vi "MicroStruct-XY-abs.vi"() -> ()   [LabVIEW 2014]
doc: "Newport Motion Controler\nThis program make lines structure\n\nAndré Romero - 2020\nandretec@ifsc.usp.br"
uses:
  <vilib>/Platform/TimedLoop/XDataNode/timing_clust.ctl
  <vilib>/Platform/TimedLoop/XDataNode/nitl_modes.ctl
  <vilib>/Platform/TimedLoop/XDataNode/wakeup.ctl
  Basic-VIs/Global Motor Axis.vi
  <vilib>/Platform/TimedLoop/XDataNode/XDataNode.xnode
  <userlib>/Newport ESP301/Newport ESP301.lvlib
  <vilib>/Platform/TimedLoop/XDataNode/XDNodeRunTimeDep.lvlib
panel:
  in  "Swap motor":bool
  out "XY Graph":cluster{dbl[], dbl[]}(graph)={[0.0, 0.0, 0.0345, 0.108, 0.2205, 0.3735, 0.564, 0.7665, 0.964, 1.0005, 1.0, 0.9995, 0.9995, 0.9815, 0.9225, 0.8235, 0.686, 0.505, 0.308, 0.108, -0.002, 0.0, 0.0005, 0.0, 0.012, 0.066, 0.1575, 0.2915, 0.465, 0.6645, 0.866, 1.0025, 1.0, 1.0, 0.9995, 0.9965, 0.9565, 0.8775, 0.7585, 0.6, 0.4055, 0.204, 0.006, -0.0005, 0.0005, 0.0, 0.0005, 0.0345, 0.108, 0.2215, 0.375, 0.566, 0.7675, 0.9685, 1.001, 1.0, 1.0, 0.9995, 0.9855, 0.9315, 0.8375, 0.7035, 0.5295, 0.331, 0.1305, -0.0025, 0.0, 0.0005, 0.0, 0.009, 0.0585, 0.148, 0.2765, 0.4475, 0.645, 0.8435, 1.003, 1.0005, 1.0, 0.9995, 0.999, 0.9625, 0.887, 0.773, 0.6175, 0.4265, 0.225, 0.028, -0.0005, 0.0005, 0.0, 0.0005, 0.031, 0.1025, 0.2125, 0.364, 0.55, 0.751, 0.9525, 1.001, 1.0, 1.0, 0.9995, 0.986, 0.9315, 0.8385, 0.705, 0.531, 0.3315, 0.1305, -0.002, 0.0, 0.0005, 0.0, 0.0085, 0.057, 0.146, 0.2735, 0.44, 0.6395, 0.8415, 1.003, 1.0, 1.0, 1.0, 0.9995, 0.9645, 0.891, 0.7775, 0.6255, 0.4355, 0.2345, 0.033, -0.0005, 0.0005, 0.0, 0.0, 0.0185, 0.0775, 0.1765, 0.3145, 0.4925, 0.6925, 0.895, 1.002, 1.0, 1.0, 0.9995, 0.9865, 0.933, 0.839, 0.7055, 0.535, 0.333, 0.1325, -0.0025, 0.0, 0.0005, 0.0, 0.0025, 0.043, 0.1225, 0.2425, 0.4015, 0.5945, 0.795, 0.9955, 1.0005, 1.0, 1.0, 0.9995, 0.965, 0.8915, 0.7775, 0.625, 0.4335, 0.235, 0.035, -0.0005, 0.0005, 0.0, 0.0, 0.0185, 0.078, 0.176, 0.3155, 0.4925, 0.693, 0.892, 1.002, 1.0, 1.0, 0.9995, 0.9865, 0.933, 0.8405, 0.706, 0.5345, 0.3325, 0.1335, -0.0025, 0.0, 0.0005, 0.0, 0.002, 0.043, 0.1225, 0.2415, 0.401, 0.594, 0.7955, 0.9945, 1.0005, 1.0, 0.9995, 0.9995, 0.9655, 0.891, 0.7775, 0.623, 0.431, 0.233, 0.032, 0.0, 0.0005, 0.0, 0.0], [0.0, 0.0, 0.0, 0.0, 0.0, 0.0, 0.0, 0.0, 0.0, 0.0, 0.021, 0.0825, 0.1015, 0.101, 0.1005, 0.1, 0.1, 0.1, 0.1, 0.1, 0.1, 0.104, 0.158, 0.2015, 0.2015, 0.2005, 0.2, 0.2, 0.2, 0.2, 0.2, 0.2, 0.2, 0.2425, 0.3015, 0.3015, 0.301, 0.3005, 0.3, 0.3, 0.3, 0.3, 0.3, 0.3, 0.328, 0.3975, 0.4015, 0.401, 0.4005, 0.4, 0.4, 0.4, 0.4, 0.4, 0.4, 0.411, 0.468, 0.5015, 0.501, 0.5005, 0.5, 0.5, 0.5, 0.5, 0.5, 0.5, 0.504, 0.557, 0.6015, 0.601, 0.6005, 0.6, 0.6, 0.6, 0.6, 0.6, 0.6, 0.6, 0.6365, 0.7015, 0.7015, 0.701, 0.7, 0.7, 0.7, 0.7, 0.7, 0.7, 0.7, 0.7275, 0.7955, 0.8015, 0.801, 0.8005, 0.8, 0.8, 0.8, 0.8, 0.8, 0.8, 0.8105, 0.868, 0.902, 0.9015, 0.9, 0.9, 0.9, 0.9, 0.9, 0.9, 0.9, 0.9005, 0.9485, 1.0015, 1.0015, 1.0005, 1.0, 1.0, 1.0, 0.9995, 0.9995, 1.0, 1.0, 1.0345, 1.1015, 1.1015, 1.101, 1.1, 1.1, 1.1, 1.1, 1.1, 1.1, 1.1, 1.128, 1.1865, 1.2015, 1.201, 1.2, 1.2, 1.2, 1.1995, 1.2, 1.2, 1.2, 1.207, 1.259, 1.3015, 1.3015, 1.3005, 1.3, 1.3, 1.3, 1.3, 1.3, 1.3, 1.3, 1.343, 1.4015, 1.4015, 1.4005, 1.4, 1.4, 1.4, 1.4, 1.3995, 1.3995, 1.4, 1.429, 1.4985, 1.5015, 1.5005, 1.5, 1.5, 1.5, 1.5, 1.5, 1.5, 1.5, 1.5175, 1.578, 1.6015, 1.601, 1.6005, 1.6, 1.6, 1.6, 1.6, 1.6, 1.6, 1.605, 1.659, 1.7015, 1.701, 1.7005, 1.7, 1.7, 1.7, 1.7, 1.7, 1.7, 1.7, 1.7425, 1.802, 1.8015, 1.8005, 1.8, 1.8, 1.8, 1.8, 1.8, 1.8, 1.8, 1.8295, 1.8995, 1.9015, 1.9005, 1.9, 1.9, 1.9, 1.9, 1.9, 1.8995, 1.8995, 1.918, 1.979, 2.002]}
  in  "N Cycles":i32=10 min=1
  in  "Acceleration (0 units/s²)":dbl=1.0 min=0.0 format="%#.4g"
  in  "Velocity (units/s)":dbl=1.0 min=0.0 format="%#.4g"
  in  "d (mm)":dbl=0.1
  in  "L (mm)":dbl=1.0
  out "X Position (mm)":dbl format="%.6g"
  out "Y Position (mm)":dbl=2.002 format="%.6g"
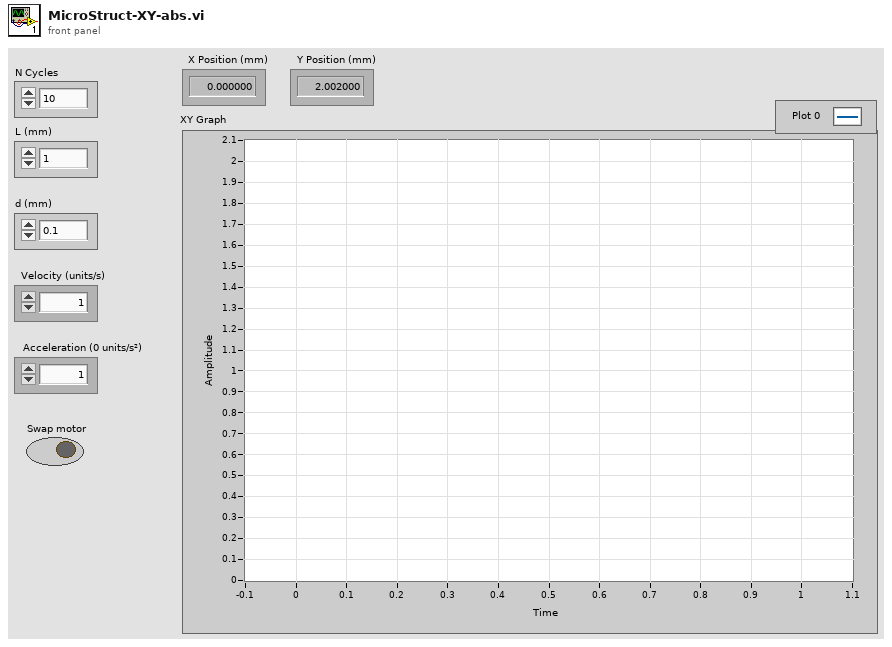
[diagram p1: front panel]
types:
  T1 = typedef "XDNodeRunTimeDep.lvlib/timing_clust.ctl" = cluster{"Expected End [f-1]":u64, "Actual End [f-1]":u64, "Finished Late? [f-1]":bool, "Expected End [i-1]":u64, "Actual End [i-1]":u64, "Finished Late? [i-1]":bool, "Expected Start [i]":u64, "Actual Start [i]":u64, "Expected Start [f]":u64, "Actual Start [f]":u64, "Source Name":string, "Structure Name":string, "Period":i64, "Deadline":i64, "Offset":i64, "Start":i64, "Priority":i32, "Timeout":i32, "Mode":T2, "Wakeup Reason":T3, "Error":errorcluster, "Source Type":string, "Secondary Source Type":string, "Global End Time":u64, "Global Start Time":u64, "Frame Duration":u64, "Iteration Duration":u64, "Assigned CPU":i32, "I/O Scan Engine Mode":u32}
  T2 = typedef "XDNodeRunTimeDep.lvlib/nitl_modes.ctl" = enum32{"No Change", "Process missed periods, maintain original phase", "Discard missed periods, maintain original phase", "Process missed periods, ignore original phase", "Discard missed periods, ignore original phase"}
  T3 = typedef "XDNodeRunTimeDep.lvlib/wakeup.ctl" = enum32{"Normal", "Aborted", "Asynchronous wakeup", "Timing source error", "Timed loop error", "Timeout"}
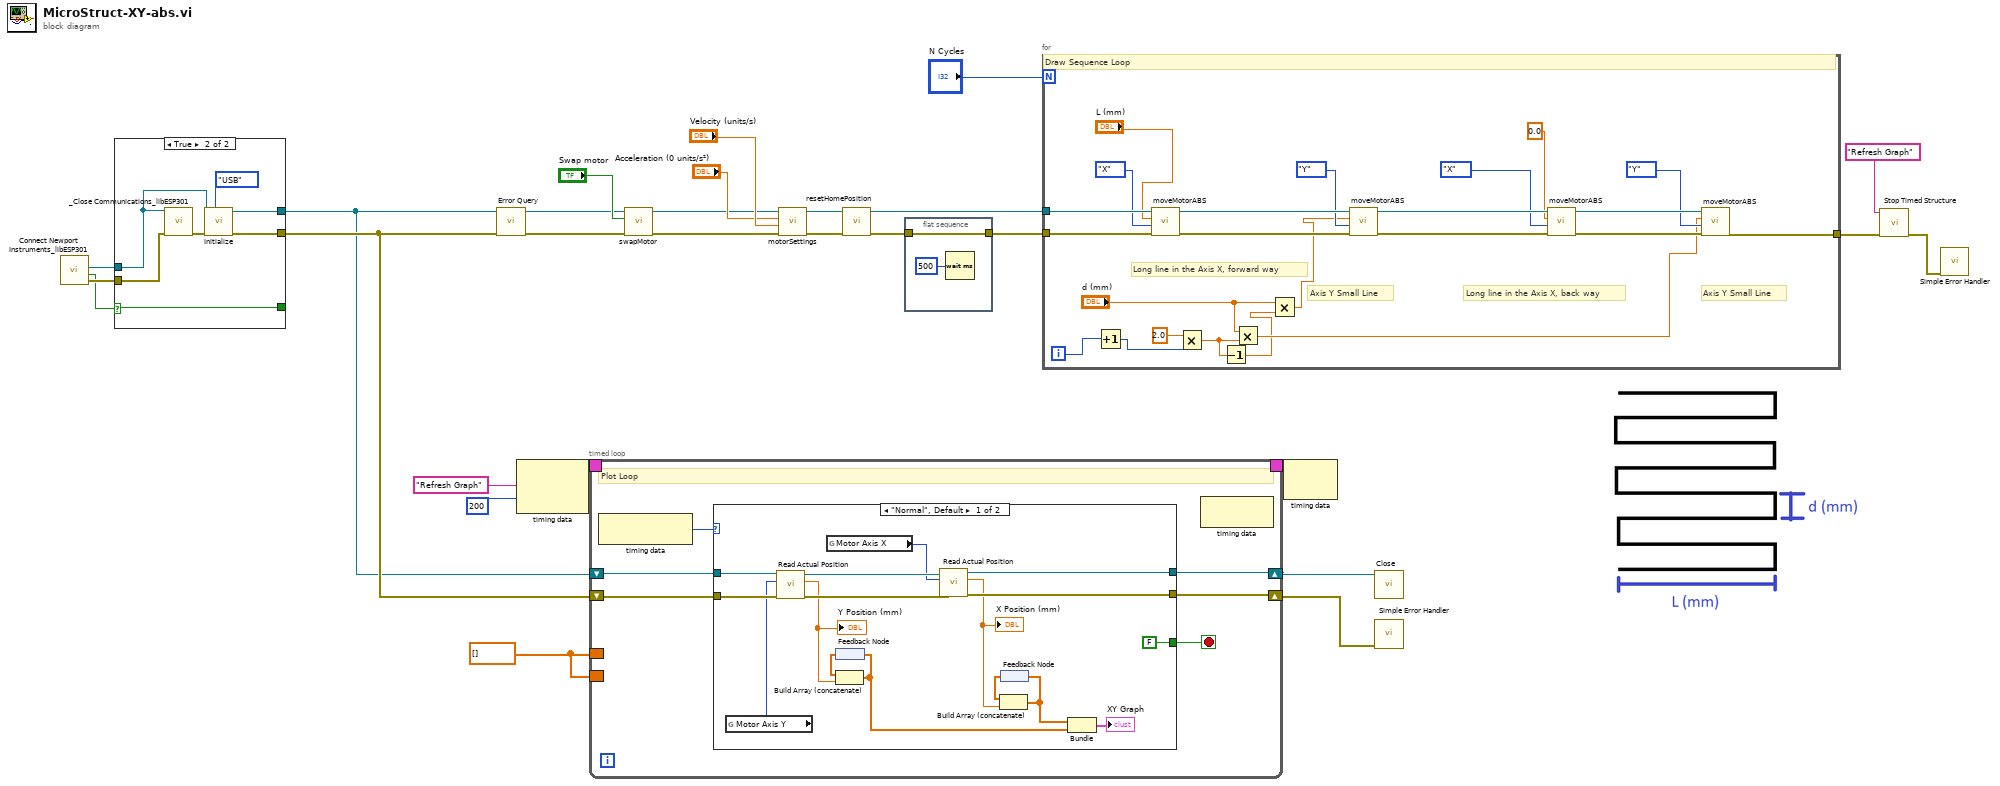
[diagram p0: block diagram]
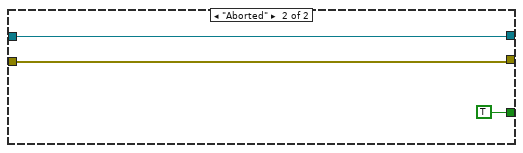
[diagram p2: hidden frame]
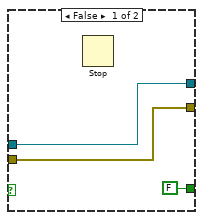
[diagram p3: hidden frame]
diagram:
  w13 = dbl[] []
  n1 = call <userlib>:"Connect Newport Instruments_libESP301.vi"() -> ("error (duplicate)"=w28:errorcluster, "Connected"=w22:bool, "VISA resource name (duplicate)"=w27:refnum<visa-resource-name>)  [unwired: 7 in, 2 out]
  n2 = case shown="True" w22 {
    selector: w22 -> [_ w32]
    tunnel: w28 -> [w29 w36]
    tunnel: w27 -> [w30 w35]
    tunnel: [w29 w34] -> w26
    tunnel: [w30 w33] -> w25
    tunnel: [FALSE w32] -> _
    frame False {
      n3 = Stop() -> ()  [unwired: 1 in]
    }
    frame True {
      n4 = call <userlib>:"_Close Communications_libESP301.vi"("Instrument Channel"=w35, "error in (no error)"=w36) -> ("error out"=w38:errorcluster)  [unwired: 13 in]
      n5 = call <userlib>:"Initialize.vi"("VISA resource name"=w35, "error in (no error)"=w38, "Serial Link (RS232)"=enum16{"RS232", "USB"}."USB") -> ("VISA resource name out"=w33:refnum<visa-resource-name>, "error out"=w34:errorcluster)  [unwired: 6 in]
    }
  }
  n6 = call <userlib>:"Error Query.vi"("error in (no error)"=w26, "VISA resource name"=w25) -> ("error out"=w8:errorcluster, "VISA resource name out"=w9:refnum<visa-resource-name>)  [unwired: 2 in, 2 out]
  n7 = node-c288("Refresh Graph" ("Structure Name"), i64 200 ("Period")) -> (w21:T1)
  n8 = timed-loop {
    timing: w21 -> [_]
    timing-out: [_] -> w20
    shift-right: [w42] -> w24
    shift-left: w25 -> [w44]
    shift-right: [w41] -> w23
    shift-left: w26 -> [w43]
    border: w13 -> [_]
    border: w13 -> [_]
    stop <- w39 stop-if-true
    # "Plot Loop"
    n9 = node-c288() -> (w40:T3)  [unwired: 1 in]
    n10 = case shown="\"Normal\", Default" w40 {
      tunnel: w44 -> [w60 w62]
      tunnel: w43 -> [w59 w61]
      tunnel: [w56 w62] -> w42
      tunnel: [w55 w61] -> w41
      tunnel: [FALSE TRUE] -> w39
      frame "Normal", Default {
        n11 = global read "Global Motor Axis.vi" "Motor Axis Y"() -> (w45:i32)
        n12 = call <userlib>:"Read Actual Position.vi"("error in (no error)"=w59, "Axis (1)"=w45, "VISA resource name"=w60) -> ("error out"=w57:errorcluster, "Position (units)"=w50:dbl, "VISA resource name out"=w58:refnum<visa-resource-name>)  [unwired: 2 in]
        "Y Position (mm)" <- w50
        n13 = global read "Global Motor Axis.vi" "Motor Axis X"() -> (w46:i32)
        n14 = feedback #1() -> (w53:dbl[])
        n15 = Build Array (concatenate)(w53, w50) -> (w48:dbl[])
        n16 = feedback-in #1(w48) -> ()
        n17 = call <userlib>:"Read Actual Position.vi"("error in (no error)"=w57, "Axis (1)"=w46, "VISA resource name"=w58) -> ("error out"=w55:errorcluster, "Position (units)"=w51:dbl, "VISA resource name out"=w56:refnum<visa-resource-name>)  [unwired: 2 in]
        "X Position (mm)" <- w51
        n18 = feedback #2() -> (w52:dbl[])
        n19 = Build Array (concatenate)(w52, w51) -> (w49:dbl[])
        n20 = feedback-in #2(w49) -> ()
        n21 = Bundle(w49, w48) -> (→"XY Graph":cluster{dbl[], dbl[]})  [unwired: 1 in]
      }
      frame "Aborted" {
      }
    }
    n22 = node-c288() -> ()  [unwired: 1 in, 1 out]
  }
  n23 = call "swapMotor.vi"("error in (no error)"=w8, "Swap motor"="Swap motor", "VISA Refnum in"=w9) -> ("error out"=w6:errorcluster, "VISA Refnum out"=w7:refnum<visa-resource-name>)  [unwired: 7 in]
  n24 = call "motorSettings.vi"("error in (no error)"=w6, "Velocity (units/s)"="Velocity (units/s)", "Acceleration (0 units/s²)"="Acceleration (0 units/s²)", "VISA Refnum in"=w7) -> ("error out"=w3:errorcluster, "VISA Refnum out"=w5:refnum<visa-resource-name>)  [unwired: 6 in]
  n25 = call "resetHomePosition.vi"("error in (no error)"=w3, "VISA Refnum in"=w5) -> ("error out"=w2:errorcluster, "VISA Refnum out"=w4:refnum<visa-resource-name>)  [unwired: 8 in]
  n26 = flat-sequence {
    tunnel: w2 -> [w68]
    tunnel: [w68] -> w1
    frame #0 {
      n27 = Wait (ms)(milliseconds to wait=u32 500) -> ()  [unwired: 1 out]
    }
  }
  n28 = for {
    N: "N Cycles" -> [_]
    tunnel: w4 -> [w91]
    tunnel: w1 -> [w90]
    tunnel: [w78] -> w12
    i -> [w77]
    # "Axis Y Small Line"
    # "Long line in the Axis X, back way"
    # "Axis Y Small Line"
    # "Long line in the Axis X, forward way"
    # "Draw Sequence Loop"
    n29 = Increment(x=w77) -> (x+1=w75:i32)
    n30 = call "moveMotorABS.vi"("error in (no error)"=w90, "Axis"=enum16{"X", "Y"}."X", "L (mm)"="L (mm)", "VISA Refnum in"=w91) -> ("error out"=w87:errorcluster, "VISA Refnum out"=w88:refnum<visa-resource-name>)  [unwired: 6 in]
    n31 = Multiply(x=2.0, y=w75) -> (x*y=w73:dbl)
    n32 = Decrement(x=w73) -> (x-1=w71:dbl)
    n33 = Multiply(x="d (mm)", y=w73) -> (x*y=w74:dbl)
    n34 = Multiply(x="d (mm)", y=w71) -> (x*y=w70:dbl)
    n35 = call "moveMotorABS.vi"("error in (no error)"=w87, "Axis"=enum16{"X", "Y"}."Y", "L (mm)"=w70, "VISA Refnum in"=w88) -> ("error out"=w84:errorcluster, "VISA Refnum out"=w85:refnum<visa-resource-name>)  [unwired: 6 in]
    n36 = call "moveMotorABS.vi"("error in (no error)"=w84, "Axis"=enum16{"X", "Y"}."X", "L (mm)"=0.0, "VISA Refnum in"=w85) -> ("error out"=w81:errorcluster, "VISA Refnum out"=w82:refnum<visa-resource-name>)  [unwired: 6 in]
    n37 = call "moveMotorABS.vi"("error in (no error)"=w81, "Axis"=enum16{"X", "Y"}."Y", "L (mm)"=w74, "VISA Refnum in"=w82) -> ("error out"=w78:errorcluster)  [unwired: 6 in, 1 out]
  }
  n38 = node-c288(w20) -> ()  [unwired: 1 out]
  n39 = call <userlib>:"Close.vi"("VISA resource name"=w24) -> ()  [unwired: 10 in, 1 out]
  n40 = call <vilib>:"Simple Error Handler.vi"("error in (no error)"=w23) -> ()  [unwired: 1 in, 8 out]
  n41 = call <vilib>:"Stop Timed Structure.vi"("error in (no error)"=w12, "name"="Refresh Graph" ("Structure Name")) -> ("error out"=w11:errorcluster)  [unwired: 9 in]
  n42 = call <vilib>:"Simple Error Handler.vi"("error in (no error)"=w11) -> ()  [unwired: 4 in, 5 out]
